vi "main(Test DQMH modules).vi"() -> ()   [LabVIEW 2018, in "Application.lvlib"] (continued)
        n3888 = Or(x=w8878, y=w8876) -> (x .or. y?=w8877:bool)
        n3889 = case shown="False" w8877 {
          tunnel: [w8906 _] -> w8888
          tunnel: w8885 -> [w8905 _]
          frame False {
            w8894 = T9 {"command"="", "data"=variant} ("element")
            w8893 = "MEAS.mux6_1"
            n3890 = To Variant(anything=T2."mux6_1_channel6_2" ("mux6_1(3wires)_encode")) -> (Variant=w8901:variant)
            n3891 = To Variant(anything=T2."mux6_1_channel6_3" ("mux6_1(3wires)_encode")) -> (Variant=w8903:variant)
            n3892 = Bundle By Name(cluster=w8894, "command"=w8893, "data"=w8901) -> (w8900:T9)
            n3893 = Bundle By Name(cluster=w8894, "command"=w8893, "data"=w8903) -> (w8899:T9)
            n3894 = Bundle By Name(cluster=w8894, "command"="MEAS.DMM dual read") -> (w8897:T9)
            n3895 = Build Array(w8900, w8899, w8897) -> (w8895:T9[])
            n3896 = Reverse 1D Array(array=w8895) -> (reversed array=w8896:T9[])
            n3897 = for {
              tunnel: [w8912] -> w8906 mode=indexing
              tunnel: w8905 -> [w8911]
              tunnel: w8896 -> [w8910] mode=indexing
              n3898 = Unbundle By Name(w8910) -> ("command"=w8909:string, "data"=w8908:variant)
              n3899 = call "App enquece.vi"("Priority Enquece"=TRUE, "command data"=w8908, "command"=w8909, "queue in"=w8911) -> ("error out"=w8912:errorcluster)  [unwired: 6 in, 1 out]
            }
          }
          frame True {
          }
        }
        n3900 = Merge Errors(w8886, w8888) -> (w8887:errorcluster)
      }
      frame "Test DRV 37" {
        w8921 = 37  # DUT index(1-60)
        n3901 = call "progress string(SubVI).vi"("String 3"=w8922, "String in"=w8923) -> ("String out"=w8924:string)  [unwired: 9 in]
        n3902 = disable-structure shown="LOGGING==TRUE" {
          disable-tunnel: w8922 -> [w8955 _]
          frame condition #0 (active) {
            n3903 = Empty String/Path?(string/path=w8955) -> (empty?=w8957:bool)
            n3904 = Select(t="Quece timeout", s=w8957, f=w8955) -> (s? t:f=w8954:string)
            n3905 = call "string log (SubVI).vi"("state Name"=w8954) -> ()  [unwired: 9 in, 2 out]
          }
          frame condition #1 {
          }
        }
        n3906 = call "FGV DRV stand.vi"() -> ("Sub-Test.DCV"=w8920:bool)  [unwired: 10 in, 1 out]
        n3907 = Not(x=w8920) -> (.not. x?=w8917:bool)
        n3908 = call "FGV Driver Data.vi"("DUT index(1-60)"=w8921) -> ("DUT SC"=w8919:bool)  [unwired: 7 in, 3 out]
        n3909 = Or(x=w8919, y=w8917) -> (x .or. y?=w8918:bool)
        n3910 = case shown="False" w8918 {
          tunnel: [w8947 _] -> w8929
          tunnel: w8926 -> [w8946 _]
          frame False {
            w8935 = T9 {"command"="", "data"=variant} ("element")
            w8934 = "MEAS.mux6_1"
            n3911 = To Variant(anything=T2."mux6_1_channel1_3" ("mux6_1(3wires)_encode")) -> (Variant=w8944:variant)
            n3912 = To Variant(anything=T2."mux6-1_channel1_2" ("mux6_1(3wires)_encode")) -> (Variant=w8942:variant)
            n3913 = Bundle By Name(cluster=w8935, "command"=w8934, "data"=w8942) -> (w8941:T9)
            n3914 = Bundle By Name(cluster=w8935, "command"=w8934, "data"=w8944) -> (w8940:T9)
            n3915 = Bundle By Name(cluster=w8935, "command"="MEAS.DMM dual read") -> (w8938:T9)
            n3916 = Build Array(w8941, w8940, w8938) -> (w8936:T9[])
            n3917 = Reverse 1D Array(array=w8936) -> (reversed array=w8937:T9[])
            n3918 = for {
              tunnel: [w8953] -> w8947 mode=indexing
              tunnel: w8946 -> [w8952]
              tunnel: w8937 -> [w8951] mode=indexing
              n3919 = Unbundle By Name(w8951) -> ("command"=w8950:string, "data"=w8949:variant)
              n3920 = call "App enquece.vi"("Priority Enquece"=TRUE, "command data"=w8949, "command"=w8950, "queue in"=w8952) -> ("error out"=w8953:errorcluster)  [unwired: 6 in, 1 out]
            }
          }
          frame True {
          }
        }
        n3921 = Merge Errors(w8927, w8929) -> (w8928:errorcluster)
      }
      frame "Test DRV 38" {
        w8963 = 38  # DUT index(1-60)
        n3922 = disable-structure shown="LOGGING==TRUE" {
          disable-tunnel: w8964 -> [w8996 _]
          frame condition #0 (active) {
            n3923 = Empty String/Path?(string/path=w8996) -> (empty?=w8998:bool)
            n3924 = Select(t="Quece timeout", s=w8998, f=w8996) -> (s? t:f=w8995:string)
            n3925 = call "string log (SubVI).vi"("state Name"=w8995) -> ()  [unwired: 9 in, 2 out]
          }
          frame condition #1 {
          }
        }
        n3926 = call "progress string(SubVI).vi"("String 3"=w8964, "String in"=w8965) -> ("String out"=w8966:string)  [unwired: 9 in]
        n3927 = call "FGV DRV stand.vi"() -> ("Sub-Test.DCV"=w8961:bool)  [unwired: 10 in, 1 out]
        n3928 = call "FGV Driver Data.vi"("DUT index(1-60)"=w8963) -> ("DUT SC"=w8960:bool)  [unwired: 7 in, 3 out]
        n3929 = Not(x=w8961) -> (.not. x?=w8958:bool)
        n3930 = Or(x=w8960, y=w8958) -> (x .or. y?=w8959:bool)
        n3931 = case shown="False" w8959 {
          tunnel: [w8988 _] -> w8970
          tunnel: w8968 -> [w8987 _]
          frame False {
            w8976 = T9 {"command"="", "data"=variant} ("element")
            w8975 = "MEAS.mux6_1"
            n3932 = To Variant(anything=T2."mux6_1_channel2_2" ("mux6_1(3wires)_encode")) -> (Variant=w8983:variant)
            n3933 = To Variant(anything=T2."mux6_1_channel2_3" ("mux6_1(3wires)_encode")) -> (Variant=w8985:variant)
            n3934 = Bundle By Name(cluster=w8976, "command"=w8975, "data"=w8983) -> (w8982:T9)
            n3935 = Bundle By Name(cluster=w8976, "command"=w8975, "data"=w8985) -> (w8981:T9)
            n3936 = Bundle By Name(cluster=w8976, "command"="MEAS.DMM dual read") -> (w8979:T9)
            n3937 = Build Array(w8982, w8981, w8979) -> (w8977:T9[])
            n3938 = Reverse 1D Array(array=w8977) -> (reversed array=w8978:T9[])
            n3939 = for {
              tunnel: [w8994] -> w8988 mode=indexing
              tunnel: w8987 -> [w8993]
              tunnel: w8978 -> [w8992] mode=indexing
              n3940 = Unbundle By Name(w8992) -> ("command"=w8991:string, "data"=w8990:variant)
              n3941 = call "App enquece.vi"("Priority Enquece"=TRUE, "command data"=w8990, "command"=w8991, "queue in"=w8993) -> ("error out"=w8994:errorcluster)  [unwired: 6 in, 1 out]
            }
          }
          frame True {
          }
        }
        n3942 = Merge Errors(w8969, w8970) -> (w8962:errorcluster)
      }
      frame "Test DRV 39" {
        w9004 = 39  # DUT index(1-60)
        n3943 = disable-structure shown="LOGGING==TRUE" {
          disable-tunnel: w9005 -> [w9037 _]
          frame condition #0 (active) {
            n3944 = Empty String/Path?(string/path=w9037) -> (empty?=w9039:bool)
            n3945 = Select(t="Quece timeout", s=w9039, f=w9037) -> (s? t:f=w9036:string)
            n3946 = call "string log (SubVI).vi"("state Name"=w9036) -> ()  [unwired: 9 in, 2 out]
          }
          frame condition #1 {
          }
        }
        n3947 = call "progress string(SubVI).vi"("String 3"=w9005, "String in"=w9006) -> ("String out"=w9007:string)  [unwired: 9 in]
        n3948 = call "FGV DRV stand.vi"() -> ("Sub-Test.DCV"=w9003:bool)  [unwired: 10 in, 1 out]
        n3949 = call "FGV Driver Data.vi"("DUT index(1-60)"=w9004) -> ("DUT SC"=w9002:bool)  [unwired: 7 in, 3 out]
        n3950 = Not(x=w9003) -> (.not. x?=w9000:bool)
        n3951 = Or(x=w9002, y=w9000) -> (x .or. y?=w9001:bool)
        n3952 = case shown="False" w9001 {
          tunnel: [w9029 _] -> w9011
          tunnel: w9009 -> [w9028 _]
          frame False {
            w9017 = T9 {"command"="", "data"=variant} ("element")
            w9016 = "MEAS.mux6_1"
            n3953 = To Variant(anything=T2."mux6_1_channel3_3" ("mux6_1(3wires)_encode")) -> (Variant=w9026:variant)
            n3954 = To Variant(anything=T2."mux6_1_channel3_2" ("mux6_1(3wires)_encode")) -> (Variant=w9024:variant)
            n3955 = Bundle By Name(cluster=w9017, "command"=w9016, "data"=w9024) -> (w9023:T9)
            n3956 = Bundle By Name(cluster=w9017, "command"=w9016, "data"=w9026) -> (w9022:T9)
            n3957 = Bundle By Name(cluster=w9017, "command"="MEAS.DMM dual read") -> (w9020:T9)
            n3958 = Build Array(w9023, w9022, w9020) -> (w9018:T9[])
            n3959 = Reverse 1D Array(array=w9018) -> (reversed array=w9019:T9[])
            n3960 = for {
              tunnel: [w9035] -> w9029 mode=indexing
              tunnel: w9028 -> [w9034]
              tunnel: w9019 -> [w9033] mode=indexing
              n3961 = Unbundle By Name(w9033) -> ("command"=w9032:string, "data"=w9031:variant)
              n3962 = call "App enquece.vi"("Priority Enquece"=TRUE, "command data"=w9031, "command"=w9032, "queue in"=w9034) -> ("error out"=w9035:errorcluster)  [unwired: 6 in, 1 out]
            }
          }
          frame True {
          }
        }
        n3963 = Merge Errors(w9010, w9011) -> (w8999:errorcluster)
      }
      frame "Test DRV 40" {
        w9044 = 40  # DUT index(1-60)
        n3964 = disable-structure shown="LOGGING==TRUE" {
          disable-tunnel: w9045 -> [w9078 _]
          frame condition #0 (active) {
            n3965 = Empty String/Path?(string/path=w9078) -> (empty?=w9080:bool)
            n3966 = Select(t="Quece timeout", s=w9080, f=w9078) -> (s? t:f=w9077:string)
            n3967 = call "string log (SubVI).vi"("state Name"=w9077) -> ()  [unwired: 9 in, 2 out]
          }
          frame condition #1 {
          }
        }
        n3968 = call "progress string(SubVI).vi"("String 3"=w9045, "String in"=w9046) -> ("String out"=w9047:string)  [unwired: 9 in]
        n3969 = call "FGV DRV stand.vi"() -> ("Sub-Test.DCV"=w9043:bool)  [unwired: 10 in, 1 out]
        n3970 = call "FGV Driver Data.vi"("DUT index(1-60)"=w9044) -> ("DUT SC"=w9042:bool)  [unwired: 7 in, 3 out]
        n3971 = Not(x=w9043) -> (.not. x?=w9040:bool)
        n3972 = Or(x=w9042, y=w9040) -> (x .or. y?=w9041:bool)
        n3973 = case shown="False" w9041 {
          tunnel: [w9070 _] -> w9052
          tunnel: w9049 -> [w9069 _]
          frame False {
            w9058 = T9 {"command"="", "data"=variant} ("element")
            w9057 = "MEAS.mux6_1"
            n3974 = To Variant(anything=T2."mux6_1_channel4_3" ("mux6_1(3wires)_encode")) -> (Variant=w9067:variant)
            n3975 = To Variant(anything=T2."mux6_1_channel4_2" ("mux6_1(3wires)_encode")) -> (Variant=w9065:variant)
            n3976 = Bundle By Name(cluster=w9058, "command"=w9057, "data"=w9065) -> (w9064:T9)
            n3977 = Bundle By Name(cluster=w9058, "command"=w9057, "data"=w9067) -> (w9063:T9)
            n3978 = Bundle By Name(cluster=w9058, "command"="MEAS.DMM dual read") -> (w9061:T9)
            n3979 = Build Array(w9064, w9063, w9061) -> (w9059:T9[])
            n3980 = Reverse 1D Array(array=w9059) -> (reversed array=w9060:T9[])
            n3981 = for {
              tunnel: [w9076] -> w9070 mode=indexing
              tunnel: w9069 -> [w9075]
              tunnel: w9060 -> [w9074] mode=indexing
              n3982 = Unbundle By Name(w9074) -> ("command"=w9073:string, "data"=w9072:variant)
              n3983 = call "App enquece.vi"("Priority Enquece"=TRUE, "command data"=w9072, "command"=w9073, "queue in"=w9075) -> ("error out"=w9076:errorcluster)  [unwired: 6 in, 1 out]
            }
          }
          frame True {
          }
        }
        n3984 = Merge Errors(w9050, w9052) -> (w9051:errorcluster)
      }
      frame "Test DRV 41" {
        w9085 = 41  # DUT index(1-60)
        n3985 = disable-structure shown="LOGGING==TRUE" {
          disable-tunnel: w9086 -> [w9119 _]
          frame condition #0 (active) {
            n3986 = Empty String/Path?(string/path=w9119) -> (empty?=w9121:bool)
            n3987 = Select(t="Quece timeout", s=w9121, f=w9119) -> (s? t:f=w9118:string)
            n3988 = call "string log (SubVI).vi"("state Name"=w9118) -> ()  [unwired: 9 in, 2 out]
          }
          frame condition #1 {
          }
        }
        n3989 = call "progress string(SubVI).vi"("String 3"=w9086, "String in"=w9087) -> ("String out"=w9088:string)  [unwired: 9 in]
        n3990 = call "FGV DRV stand.vi"() -> ("Sub-Test.DCV"=w9084:bool)  [unwired: 10 in, 1 out]
        n3991 = call "FGV Driver Data.vi"("DUT index(1-60)"=w9085) -> ("DUT SC"=w9083:bool)  [unwired: 7 in, 3 out]
        n3992 = Not(x=w9084) -> (.not. x?=w9081:bool)
        n3993 = Or(x=w9083, y=w9081) -> (x .or. y?=w9082:bool)
        n3994 = case shown="False" w9082 {
          tunnel: [w9111 _] -> w9093
          tunnel: w9090 -> [w9110 _]
          frame False {
            w9099 = T9 {"command"="", "data"=variant} ("element")
            w9098 = "MEAS.mux6_1"
            n3995 = To Variant(anything=T2."mux6_1_channel5_3" ("mux6_1(3wires)_encode")) -> (Variant=w9108:variant)
            n3996 = To Variant(anything=T2."mux6_1_channel5_2" ("mux6_1(3wires)_encode")) -> (Variant=w9106:variant)
            n3997 = Bundle By Name(cluster=w9099, "command"=w9098, "data"=w9106) -> (w9105:T9)
            n3998 = Bundle By Name(cluster=w9099, "command"=w9098, "data"=w9108) -> (w9104:T9)
            n3999 = Bundle By Name(cluster=w9099, "command"="MEAS.DMM dual read") -> (w9102:T9)
            n4000 = Build Array(w9105, w9104, w9102) -> (w9100:T9[])
            n4001 = Reverse 1D Array(array=w9100) -> (reversed array=w9101:T9[])
            n4002 = for {
              tunnel: [w9117] -> w9111 mode=indexing
              tunnel: w9110 -> [w9116]
              tunnel: w9101 -> [w9115] mode=indexing
              n4003 = Unbundle By Name(w9115) -> ("command"=w9114:string, "data"=w9113:variant)
              n4004 = call "App enquece.vi"("Priority Enquece"=TRUE, "command data"=w9113, "command"=w9114, "queue in"=w9116) -> ("error out"=w9117:errorcluster)  [unwired: 6 in, 1 out]
            }
          }
          frame True {
          }
        }
        n4005 = Merge Errors(w9091, w9093) -> (w9092:errorcluster)
      }
      frame "Test DRV 42" {
        w9126 = 42  # DUT index(1-60)
        n4006 = disable-structure shown="LOGGING==TRUE" {
          disable-tunnel: w9127 -> [w9160 _]
          frame condition #0 (active) {
            n4007 = Empty String/Path?(string/path=w9160) -> (empty?=w9162:bool)
            n4008 = Select(t="Quece timeout", s=w9162, f=w9160) -> (s? t:f=w9159:string)
            n4009 = call "string log (SubVI).vi"("state Name"=w9159) -> ()  [unwired: 9 in, 2 out]
          }
          frame condition #1 {
          }
        }
        n4010 = call "progress string(SubVI).vi"("String 3"=w9127, "String in"=w9128) -> ("String out"=w9129:string)  [unwired: 9 in]
        n4011 = call "FGV DRV stand.vi"() -> ("Sub-Test.DCV"=w9125:bool)  [unwired: 10 in, 1 out]
        n4012 = call "FGV Driver Data.vi"("DUT index(1-60)"=w9126) -> ("DUT SC"=w9124:bool)  [unwired: 7 in, 3 out]
        n4013 = Not(x=w9125) -> (.not. x?=w9122:bool)
        n4014 = Or(x=w9124, y=w9122) -> (x .or. y?=w9123:bool)
        n4015 = case shown="False" w9123 {
          tunnel: [w9152 _] -> w9134
          tunnel: w9131 -> [w9151 _]
          frame False {
            w9140 = T9 {"command"="", "data"=variant} ("element")
            w9139 = "MEAS.mux6_1"
            n4016 = To Variant(anything=T2."mux6_1_channel6_3" ("mux6_1(3wires)_encode")) -> (Variant=w9149:variant)
            n4017 = To Variant(anything=T2."mux6_1_channel6_2" ("mux6_1(3wires)_encode")) -> (Variant=w9147:variant)
            n4018 = Bundle By Name(cluster=w9140, "command"=w9139, "data"=w9147) -> (w9146:T9)
            n4019 = Bundle By Name(cluster=w9140, "command"=w9139, "data"=w9149) -> (w9145:T9)
            n4020 = Bundle By Name(cluster=w9140, "command"="MEAS.DMM dual read") -> (w9143:T9)
            n4021 = Build Array(w9146, w9145, w9143) -> (w9141:T9[])
            n4022 = Reverse 1D Array(array=w9141) -> (reversed array=w9142:T9[])
            n4023 = for {
              tunnel: [w9158] -> w9152 mode=indexing
              tunnel: w9151 -> [w9153]
              tunnel: w9142 -> [w9154] mode=indexing
              n4024 = Unbundle By Name(w9154) -> ("command"=w9157:string, "data"=w9156:variant)
              n4025 = call "App enquece.vi"("Priority Enquece"=TRUE, "command data"=w9156, "command"=w9157, "queue in"=w9153) -> ("error out"=w9158:errorcluster)  [unwired: 6 in, 1 out]
            }
          }
          frame True {
          }
        }
        n4026 = Merge Errors(w9132, w9134) -> (w9133:errorcluster)
      }
      frame "Test DRV 43" {
        w9167 = 43  # DUT index(1-60)
        n4027 = disable-structure shown="LOGGING==TRUE" {
          disable-tunnel: w9168 -> [w9201 _]
          frame condition #0 (active) {
            n4028 = Empty String/Path?(string/path=w9201) -> (empty?=w9203:bool)
            n4029 = Select(t="Quece timeout", s=w9203, f=w9201) -> (s? t:f=w9200:string)
            n4030 = call "string log (SubVI).vi"("state Name"=w9200) -> ()  [unwired: 9 in, 2 out]
          }
          frame condition #1 {
          }
        }
        n4031 = call "progress string(SubVI).vi"("String 3"=w9168, "String in"=w9169) -> ("String out"=w9170:string)  [unwired: 9 in]
        n4032 = call "FGV DRV stand.vi"() -> ("Sub-Test.DCV"=w9166:bool)  [unwired: 10 in, 1 out]
        n4033 = call "FGV Driver Data.vi"("DUT index(1-60)"=w9167) -> ("DUT SC"=w9165:bool)  [unwired: 7 in, 3 out]
        n4034 = Not(x=w9166) -> (.not. x?=w9163:bool)
        n4035 = Or(x=w9165, y=w9163) -> (x .or. y?=w9164:bool)
        n4036 = case shown="False" w9164 {
          tunnel: [w9193 _] -> w9175
          tunnel: w9172 -> [w9192 _]
          frame False {
            w9181 = T9 {"command"="", "data"=variant} ("element")
            w9180 = "MEAS.mux6_1"
            n4037 = To Variant(anything=T2."mux6_1_channel1_3" ("mux6_1(3wires)_encode")) -> (Variant=w9190:variant)
            n4038 = To Variant(anything=T2."mux6-1_channel1_2" ("mux6_1(3wires)_encode")) -> (Variant=w9188:variant)
            n4039 = Bundle By Name(cluster=w9181, "command"=w9180, "data"=w9188) -> (w9187:T9)
            n4040 = Bundle By Name(cluster=w9181, "command"=w9180, "data"=w9190) -> (w9186:T9)
            n4041 = Bundle By Name(cluster=w9181, "command"="MEAS.DMM dual read") -> (w9184:T9)
            n4042 = Build Array(w9187, w9186, w9184) -> (w9182:T9[])
            n4043 = Reverse 1D Array(array=w9182) -> (reversed array=w9183:T9[])
            n4044 = for {
              tunnel: [w9199] -> w9193 mode=indexing
              tunnel: w9192 -> [w9198]
              tunnel: w9183 -> [w9197] mode=indexing
              n4045 = Unbundle By Name(w9197) -> ("command"=w9196:string, "data"=w9195:variant)
              n4046 = call "App enquece.vi"("Priority Enquece"=TRUE, "command data"=w9195, "command"=w9196, "queue in"=w9198) -> ("error out"=w9199:errorcluster)  [unwired: 6 in, 1 out]
            }
          }
          frame True {
          }
        }
        n4047 = Merge Errors(w9173, w9175) -> (w9174:errorcluster)
      }
      frame "Test DRV 44" {
        w9208 = 44  # DUT index(1-60)
        n4048 = disable-structure shown="LOGGING==TRUE" {
          disable-tunnel: w9209 -> [w9242 _]
          frame condition #0 (active) {
            n4049 = Empty String/Path?(string/path=w9242) -> (empty?=w9244:bool)
            n4050 = Select(t="Quece timeout", s=w9244, f=w9242) -> (s? t:f=w9241:string)
            n4051 = call "string log (SubVI).vi"("state Name"=w9241) -> ()  [unwired: 9 in, 2 out]
          }
          frame condition #1 {
          }
        }
        n4052 = call "progress string(SubVI).vi"("String 3"=w9209, "String in"=w9210) -> ("String out"=w9211:string)  [unwired: 9 in]
        n4053 = call "FGV DRV stand.vi"() -> ("Sub-Test.DCV"=w9207:bool)  [unwired: 10 in, 1 out]
        n4054 = call "FGV Driver Data.vi"("DUT index(1-60)"=w9208) -> ("DUT SC"=w9206:bool)  [unwired: 7 in, 3 out]
        n4055 = Not(x=w9207) -> (.not. x?=w9204:bool)
        n4056 = Or(x=w9206, y=w9204) -> (x .or. y?=w9205:bool)
        n4057 = case shown="False" w9205 {
          tunnel: [w9234 _] -> w9216
          tunnel: w9213 -> [w9233 _]
          frame False {
            w9222 = T9 {"command"="", "data"=variant} ("element")
            w9221 = "MEAS.mux6_1"
            n4058 = To Variant(anything=T2."mux6_1_channel2_3" ("mux6_1(3wires)_encode")) -> (Variant=w9231:variant)
            n4059 = To Variant(anything=T2."mux6_1_channel2_2" ("mux6_1(3wires)_encode")) -> (Variant=w9229:variant)
            n4060 = Bundle By Name(cluster=w9222, "command"=w9221, "data"=w9229) -> (w9228:T9)
            n4061 = Bundle By Name(cluster=w9222, "command"=w9221, "data"=w9231) -> (w9227:T9)
            n4062 = Bundle By Name(cluster=w9222, "command"="MEAS.DMM dual read") -> (w9225:T9)
            n4063 = Build Array(w9228, w9227, w9225) -> (w9223:T9[])
            n4064 = Reverse 1D Array(array=w9223) -> (reversed array=w9224:T9[])
            n4065 = for {
              tunnel: [w9240] -> w9234 mode=indexing
              tunnel: w9233 -> [w9239]
              tunnel: w9224 -> [w9238] mode=indexing
              n4066 = Unbundle By Name(w9238) -> ("command"=w9237:string, "data"=w9236:variant)
              n4067 = call "App enquece.vi"("Priority Enquece"=TRUE, "command data"=w9236, "command"=w9237, "queue in"=w9239) -> ("error out"=w9240:errorcluster)  [unwired: 6 in, 1 out]
            }
          }
          frame True {
          }
        }
        n4068 = Merge Errors(w9214, w9216) -> (w9215:errorcluster)
      }
      frame "Test DRV 45" {
        w9249 = 45  # DUT index(1-60)
        n4069 = disable-structure shown="LOGGING==TRUE" {
          disable-tunnel: w9250 -> [w9283 _]
          frame condition #0 (active) {
            n4070 = Empty String/Path?(string/path=w9283) -> (empty?=w9285:bool)
            n4071 = Select(t="Quece timeout", s=w9285, f=w9283) -> (s? t:f=w9282:string)
            n4072 = call "string log (SubVI).vi"("state Name"=w9282) -> ()  [unwired: 9 in, 2 out]
          }
          frame condition #1 {
          }
        }
        n4073 = call "progress string(SubVI).vi"("String 3"=w9250, "String in"=w9251) -> ("String out"=w9252:string)  [unwired: 9 in]
        n4074 = call "FGV DRV stand.vi"() -> ("Sub-Test.DCV"=w9248:bool)  [unwired: 10 in, 1 out]
        n4075 = call "FGV Driver Data.vi"("DUT index(1-60)"=w9249) -> ("DUT SC"=w9247:bool)  [unwired: 7 in, 3 out]
        n4076 = Not(x=w9248) -> (.not. x?=w9245:bool)
        n4077 = Or(x=w9247, y=w9245) -> (x .or. y?=w9246:bool)
        n4078 = case shown="False" w9246 {
          tunnel: [w9275 _] -> w9257
          tunnel: w9254 -> [w9274 _]
          frame False {
            w9263 = T9 {"command"="", "data"=variant} ("element")
            w9262 = "MEAS.mux6_1"
            n4079 = To Variant(anything=T2."mux6_1_channel3_3" ("mux6_1(3wires)_encode")) -> (Variant=w9272:variant)
            n4080 = To Variant(anything=T2."mux6_1_channel3_2" ("mux6_1(3wires)_encode")) -> (Variant=w9270:variant)
            n4081 = Bundle By Name(cluster=w9263, "command"=w9262, "data"=w9270) -> (w9269:T9)
            n4082 = Bundle By Name(cluster=w9263, "command"=w9262, "data"=w9272) -> (w9268:T9)
            n4083 = Bundle By Name(cluster=w9263, "command"="MEAS.DMM dual read") -> (w9266:T9)
            n4084 = Build Array(w9269, w9268, w9266) -> (w9264:T9[])
            n4085 = Reverse 1D Array(array=w9264) -> (reversed array=w9265:T9[])
            n4086 = for {
              tunnel: [w9281] -> w9275 mode=indexing
              tunnel: w9274 -> [w9280]
              tunnel: w9265 -> [w9279] mode=indexing
              n4087 = Unbundle By Name(w9279) -> ("command"=w9278:string, "data"=w9277:variant)
              n4088 = call "App enquece.vi"("Priority Enquece"=TRUE, "command data"=w9277, "command"=w9278, "queue in"=w9280) -> ("error out"=w9281:errorcluster)  [unwired: 6 in, 1 out]
            }
          }
          frame True {
          }
        }
        n4089 = Merge Errors(w9255, w9257) -> (w9256:errorcluster)
      }
      frame "Test DRV 46" {
        w9290 = 46  # DUT index(1-60)
        n4090 = disable-structure shown="LOGGING==TRUE" {
          disable-tunnel: w9291 -> [w9324 _]
          frame condition #0 (active) {
            n4091 = Empty String/Path?(string/path=w9324) -> (empty?=w9326:bool)
            n4092 = Select(t="Quece timeout", s=w9326, f=w9324) -> (s? t:f=w9323:string)
            n4093 = call "string log (SubVI).vi"("state Name"=w9323) -> ()  [unwired: 9 in, 2 out]
          }
          frame condition #1 {
          }
        }
        n4094 = call "progress string(SubVI).vi"("String 3"=w9291, "String in"=w9292) -> ("String out"=w9293:string)  [unwired: 9 in]
        n4095 = call "FGV DRV stand.vi"() -> ("Sub-Test.DCV"=w9289:bool)  [unwired: 10 in, 1 out]
        n4096 = call "FGV Driver Data.vi"("DUT index(1-60)"=w9290) -> ("DUT SC"=w9288:bool)  [unwired: 7 in, 3 out]
        n4097 = Not(x=w9289) -> (.not. x?=w9286:bool)
        n4098 = Or(x=w9288, y=w9286) -> (x .or. y?=w9287:bool)
        n4099 = case shown="False" w9287 {
          tunnel: [w9316 _] -> w9298
          tunnel: w9295 -> [w9315 _]
          frame False {
            w9304 = T9 {"command"="", "data"=variant} ("element")
            w9303 = "MEAS.mux6_1"
            n4100 = To Variant(anything=T2."mux6_1_channel4_3" ("mux6_1(3wires)_encode")) -> (Variant=w9313:variant)
            n4101 = To Variant(anything=T2."mux6_1_channel4_2" ("mux6_1(3wires)_encode")) -> (Variant=w9311:variant)
            n4102 = Bundle By Name(cluster=w9304, "command"=w9303, "data"=w9311) -> (w9310:T9)
            n4103 = Bundle By Name(cluster=w9304, "command"=w9303, "data"=w9313) -> (w9309:T9)
            n4104 = Bundle By Name(cluster=w9304, "command"="MEAS.DMM dual read") -> (w9307:T9)
            n4105 = Build Array(w9310, w9309, w9307) -> (w9305:T9[])
            n4106 = Reverse 1D Array(array=w9305) -> (reversed array=w9306:T9[])
            n4107 = for {
              tunnel: [w9322] -> w9316 mode=indexing
              tunnel: w9315 -> [w9321]
              tunnel: w9306 -> [w9320] mode=indexing
              n4108 = Unbundle By Name(w9320) -> ("command"=w9319:string, "data"=w9318:variant)
              n4109 = call "App enquece.vi"("Priority Enquece"=TRUE, "command data"=w9318, "command"=w9319, "queue in"=w9321) -> ("error out"=w9322:errorcluster)  [unwired: 6 in, 1 out]
            }
          }
          frame True {
          }
        }
        n4110 = Merge Errors(w9296, w9298) -> (w9297:errorcluster)
      }
      frame "Test DRV 47" {
        w9331 = 47  # DUT index(1-60)
        n4111 = disable-structure shown="LOGGING==TRUE" {
          disable-tunnel: w9332 -> [w9365 _]
          frame condition #0 (active) {
            n4112 = Empty String/Path?(string/path=w9365) -> (empty?=w9367:bool)
            n4113 = Select(t="Quece timeout", s=w9367, f=w9365) -> (s? t:f=w9364:string)
            n4114 = call "string log (SubVI).vi"("state Name"=w9364) -> ()  [unwired: 9 in, 2 out]
          }
          frame condition #1 {
          }
        }
        n4115 = call "progress string(SubVI).vi"("String 3"=w9332, "String in"=w9333) -> ("String out"=w9334:string)  [unwired: 9 in]
        n4116 = call "FGV DRV stand.vi"() -> ("Sub-Test.DCV"=w9330:bool)  [unwired: 10 in, 1 out]
        n4117 = call "FGV Driver Data.vi"("DUT index(1-60)"=w9331) -> ("DUT SC"=w9329:bool)  [unwired: 7 in, 3 out]
        n4118 = Not(x=w9330) -> (.not. x?=w9327:bool)
        n4119 = Or(x=w9329, y=w9327) -> (x .or. y?=w9328:bool)
        n4120 = case shown="False" w9328 {
          tunnel: [w9357 _] -> w9339
          tunnel: w9336 -> [w9356 _]
          frame False {
            w9345 = T9 {"command"="", "data"=variant} ("element")
            w9344 = "MEAS.mux6_1"
            n4121 = To Variant(anything=T2."mux6_1_channel5_3" ("mux6_1(3wires)_encode")) -> (Variant=w9354:variant)
            n4122 = To Variant(anything=T2."mux6_1_channel5_2" ("mux6_1(3wires)_encode")) -> (Variant=w9352:variant)
            n4123 = Bundle By Name(cluster=w9345, "command"=w9344, "data"=w9352) -> (w9351:T9)
            n4124 = Bundle By Name(cluster=w9345, "command"=w9344, "data"=w9354) -> (w9350:T9)
            n4125 = Bundle By Name(cluster=w9345, "command"="MEAS.DMM dual read") -> (w9348:T9)
            n4126 = Build Array(w9351, w9350, w9348) -> (w9346:T9[])
            n4127 = Reverse 1D Array(array=w9346) -> (reversed array=w9347:T9[])
            n4128 = for {
              tunnel: [w9363] -> w9357 mode=indexing
              tunnel: w9356 -> [w9362]
              tunnel: w9347 -> [w9361] mode=indexing
              n4129 = Unbundle By Name(w9361) -> ("command"=w9360:string, "data"=w9359:variant)
              n4130 = call "App enquece.vi"("Priority Enquece"=TRUE, "command data"=w9359, "command"=w9360, "queue in"=w9362) -> ("error out"=w9363:errorcluster)  [unwired: 6 in, 1 out]
            }
          }
          frame True {
          }
        }
        n4131 = Merge Errors(w9337, w9339) -> (w9338:errorcluster)
      }
      frame "Test DRV 48" {
        w9372 = 48  # DUT index(1-60)
        n4132 = disable-structure shown="LOGGING==TRUE" {
          disable-tunnel: w9373 -> [w9406 _]
          frame condition #0 (active) {
            n4133 = Empty String/Path?(string/path=w9406) -> (empty?=w9408:bool)
            n4134 = Select(t="Quece timeout", s=w9408, f=w9406) -> (s? t:f=w9405:string)
            n4135 = call "string log (SubVI).vi"("state Name"=w9405) -> ()  [unwired: 9 in, 2 out]
          }
          frame condition #1 {
          }
        }
        n4136 = call "progress string(SubVI).vi"("String 3"=w9373, "String in"=w9374) -> ("String out"=w9375:string)  [unwired: 9 in]
        n4137 = call "FGV DRV stand.vi"() -> ("Sub-Test.DCV"=w9371:bool)  [unwired: 10 in, 1 out]
        n4138 = call "FGV Driver Data.vi"("DUT index(1-60)"=w9372) -> ("DUT SC"=w9370:bool)  [unwired: 7 in, 3 out]
        n4139 = Not(x=w9371) -> (.not. x?=w9368:bool)
        n4140 = Or(x=w9370, y=w9368) -> (x .or. y?=w9369:bool)
        n4141 = case shown="False" w9369 {
          tunnel: [w9398 _] -> w9380
          tunnel: w9377 -> [w9397 _]
          frame False {
            w9386 = T9 {"command"="", "data"=variant} ("element")
            w9385 = "MEAS.mux6_1"
            n4142 = To Variant(anything=T2."mux6_1_channel6_3" ("mux6_1(3wires)_encode")) -> (Variant=w9395:variant)
            n4143 = To Variant(anything=T2."mux6_1_channel6_2" ("mux6_1(3wires)_encode")) -> (Variant=w9393:variant)
            n4144 = Bundle By Name(cluster=w9386, "command"=w9385, "data"=w9393) -> (w9392:T9)
            n4145 = Bundle By Name(cluster=w9386, "command"=w9385, "data"=w9395) -> (w9391:T9)
            n4146 = Bundle By Name(cluster=w9386, "command"="MEAS.DMM dual read") -> (w9389:T9)
            n4147 = Build Array(w9392, w9391, w9389) -> (w9387:T9[])
            n4148 = Reverse 1D Array(array=w9387) -> (reversed array=w9388:T9[])
            n4149 = for {
              tunnel: [w9404] -> w9398 mode=indexing
              tunnel: w9397 -> [w9403]
              tunnel: w9388 -> [w9402] mode=indexing
              n4150 = Unbundle By Name(w9402) -> ("command"=w9401:string, "data"=w9400:variant)
              n4151 = call "App enquece.vi"("Priority Enquece"=TRUE, "command data"=w9400, "command"=w9401, "queue in"=w9403) -> ("error out"=w9404:errorcluster)  [unwired: 6 in, 1 out]
            }
          }
          frame True {
          }
        }
        n4152 = Merge Errors(w9378, w9380) -> (w9379:errorcluster)
      }
      frame "Test DRV 49" {
        w9413 = 49  # DUT index(1-60)
        n4153 = disable-structure shown="LOGGING==TRUE" {
          disable-tunnel: w9414 -> [w9447 _]
          frame condition #0 (active) {
            n4154 = Empty String/Path?(string/path=w9447) -> (empty?=w9449:bool)
            n4155 = Select(t="Quece timeout", s=w9449, f=w9447) -> (s? t:f=w9446:string)
            n4156 = call "string log (SubVI).vi"("state Name"=w9446) -> ()  [unwired: 9 in, 2 out]
          }
          frame condition #1 {
          }
        }
        n4157 = call "progress string(SubVI).vi"("String 3"=w9414, "String in"=w9415) -> ("String out"=w9416:string)  [unwired: 9 in]
        n4158 = call "FGV DRV stand.vi"() -> ("Sub-Test.DCV"=w9412:bool)  [unwired: 10 in, 1 out]
        n4159 = call "FGV Driver Data.vi"("DUT index(1-60)"=w9413) -> ("DUT SC"=w9411:bool)  [unwired: 7 in, 3 out]
        n4160 = Not(x=w9412) -> (.not. x?=w9409:bool)
        n4161 = Or(x=w9411, y=w9409) -> (x .or. y?=w9410:bool)
        n4162 = case shown="False" w9410 {
          tunnel: [w9439 _] -> w9421
          tunnel: w9418 -> [w9438 _]
          frame False {
            w9427 = T9 {"command"="", "data"=variant} ("element")
            w9426 = "MEAS.mux6_1"
            n4163 = To Variant(anything=T2."mux6_1_channel1_3" ("mux6_1(3wires)_encode")) -> (Variant=w9436:variant)
            n4164 = To Variant(anything=T2."mux6-1_channel1_2" ("mux6_1(3wires)_encode")) -> (Variant=w9434:variant)
            n4165 = Bundle By Name(cluster=w9427, "command"=w9426, "data"=w9434) -> (w9433:T9)
            n4166 = Bundle By Name(cluster=w9427, "command"=w9426, "data"=w9436) -> (w9432:T9)
            n4167 = Bundle By Name(cluster=w9427, "command"="MEAS.DMM dual read") -> (w9430:T9)
            n4168 = Build Array(w9433, w9432, w9430) -> (w9428:T9[])
            n4169 = Reverse 1D Array(array=w9428) -> (reversed array=w9429:T9[])
            n4170 = for {
              tunnel: [w9445] -> w9439 mode=indexing
              tunnel: w9438 -> [w9444]
              tunnel: w9429 -> [w9443] mode=indexing
              n4171 = Unbundle By Name(w9443) -> ("command"=w9442:string, "data"=w9441:variant)
              n4172 = call "App enquece.vi"("Priority Enquece"=TRUE, "command data"=w9441, "command"=w9442, "queue in"=w9444) -> ("error out"=w9445:errorcluster)  [unwired: 6 in, 1 out]
            }
          }
          frame True {
          }
        }
        n4173 = Merge Errors(w9419, w9421) -> (w9420:errorcluster)
      }
      frame "Test DRV 50" {
        w9454 = 50  # DUT index(1-60)
        n4174 = disable-structure shown="LOGGING==TRUE" {
          disable-tunnel: w9455 -> [w9488 _]
          frame condition #0 (active) {
            n4175 = Empty String/Path?(string/path=w9488) -> (empty?=w9490:bool)
            n4176 = Select(t="Quece timeout", s=w9490, f=w9488) -> (s? t:f=w9487:string)
            n4177 = call "string log (SubVI).vi"("state Name"=w9487) -> ()  [unwired: 9 in, 2 out]
          }
          frame condition #1 {
          }
        }
        n4178 = call "progress string(SubVI).vi"("String 3"=w9455, "String in"=w9456) -> ("String out"=w9457:string)  [unwired: 9 in]
        n4179 = call "FGV DRV stand.vi"() -> ("Sub-Test.DCV"=w9453:bool)  [unwired: 10 in, 1 out]
        n4180 = call "FGV Driver Data.vi"("DUT index(1-60)"=w9454) -> ("DUT SC"=w9452:bool)  [unwired: 7 in, 3 out]
        n4181 = Not(x=w9453) -> (.not. x?=w9450:bool)
        n4182 = Or(x=w9452, y=w9450) -> (x .or. y?=w9451:bool)
        n4183 = case shown="False" w9451 {
          tunnel: [w9480 _] -> w9462
          tunnel: w9459 -> [w9467 _]
          frame False {
            w9469 = T9 {"command"="", "data"=variant} ("element")
            w9468 = "MEAS.mux6_1"
            n4184 = To Variant(anything=T2."mux6_1_channel2_3" ("mux6_1(3wires)_encode")) -> (Variant=w9478:variant)
            n4185 = To Variant(anything=T2."mux6_1_channel2_2" ("mux6_1(3wires)_encode")) -> (Variant=w9476:variant)
            n4186 = Bundle By Name(cluster=w9469, "command"=w9468, "data"=w9476) -> (w9475:T9)
            n4187 = Bundle By Name(cluster=w9469, "command"=w9468, "data"=w9478) -> (w9474:T9)
            n4188 = Bundle By Name(cluster=w9469, "command"="MEAS.DMM dual read") -> (w9472:T9)
            n4189 = Build Array(w9475, w9474, w9472) -> (w9470:T9[])
            n4190 = Reverse 1D Array(array=w9470) -> (reversed array=w9471:T9[])
            n4191 = for {
              tunnel: [w9486] -> w9480 mode=indexing
              tunnel: w9467 -> [w9485]
              tunnel: w9471 -> [w9484] mode=indexing
              n4192 = Unbundle By Name(w9484) -> ("command"=w9483:string, "data"=w9482:variant)
              n4193 = call "App enquece.vi"("Priority Enquece"=TRUE, "command data"=w9482, "command"=w9483, "queue in"=w9485) -> ("error out"=w9486:errorcluster)  [unwired: 6 in, 1 out]
            }
          }
          frame True {
          }
        }
        n4194 = Merge Errors(w9460, w9462) -> (w9461:errorcluster)
      }
      frame "Test DRV 51" {
        w9495 = 51  # DUT index(1-60)
        n4195 = disable-structure shown="LOGGING==TRUE" {
          disable-tunnel: w9496 -> [w9529 _]
          frame condition #0 (active) {
            n4196 = Empty String/Path?(string/path=w9529) -> (empty?=w9531:bool)
            n4197 = Select(t="Quece timeout", s=w9531, f=w9529) -> (s? t:f=w9528:string)
            n4198 = call "string log (SubVI).vi"("state Name"=w9528) -> ()  [unwired: 9 in, 2 out]
          }
          frame condition #1 {
          }
        }
        n4199 = call "progress string(SubVI).vi"("String 3"=w9496, "String in"=w9497) -> ("String out"=w9498:string)  [unwired: 9 in]
        n4200 = call "FGV DRV stand.vi"() -> ("Sub-Test.DCV"=w9494:bool)  [unwired: 10 in, 1 out]
        n4201 = call "FGV Driver Data.vi"("DUT index(1-60)"=w9495) -> ("DUT SC"=w9493:bool)  [unwired: 7 in, 3 out]
        n4202 = Not(x=w9494) -> (.not. x?=w9491:bool)
        n4203 = Or(x=w9493, y=w9491) -> (x .or. y?=w9492:bool)
        n4204 = case shown="False" w9492 {
          tunnel: [w9521 _] -> w9503
          tunnel: w9500 -> [w9520 _]
          frame False {
            w9509 = T9 {"command"="", "data"=variant} ("element")
            w9508 = "MEAS.mux6_1"
            n4205 = To Variant(anything=T2."mux6_1_channel3_3" ("mux6_1(3wires)_encode")) -> (Variant=w9518:variant)
            n4206 = To Variant(anything=T2."mux6_1_channel3_2" ("mux6_1(3wires)_encode")) -> (Variant=w9516:variant)
            n4207 = Bundle By Name(cluster=w9509, "command"=w9508, "data"=w9516) -> (w9515:T9)
            n4208 = Bundle By Name(cluster=w9509, "command"=w9508, "data"=w9518) -> (w9514:T9)
            n4209 = Bundle By Name(cluster=w9509, "command"="MEAS.DMM dual read") -> (w9512:T9)
            n4210 = Build Array(w9515, w9514, w9512) -> (w9510:T9[])
            n4211 = Reverse 1D Array(array=w9510) -> (reversed array=w9511:T9[])
            n4212 = for {
              tunnel: [w9527] -> w9521 mode=indexing
              tunnel: w9520 -> [w9526]
              tunnel: w9511 -> [w9525] mode=indexing
              n4213 = Unbundle By Name(w9525) -> ("command"=w9524:string, "data"=w9523:variant)
              n4214 = call "App enquece.vi"("Priority Enquece"=TRUE, "command data"=w9523, "command"=w9524, "queue in"=w9526) -> ("error out"=w9527:errorcluster)  [unwired: 6 in, 1 out]
            }
          }
          frame True {
          }
        }
        n4215 = Merge Errors(w9501, w9503) -> (w9502:errorcluster)
      }
      frame "Test DRV 52" {
        w9536 = 52  # DUT index(1-60)
        n4216 = disable-structure shown="LOGGING==TRUE" {
          disable-tunnel: w9537 -> [w9570 _]
          frame condition #0 (active) {
            n4217 = Empty String/Path?(string/path=w9570) -> (empty?=w9572:bool)
            n4218 = Select(t="Quece timeout", s=w9572, f=w9570) -> (s? t:f=w9569:string)
            n4219 = call "string log (SubVI).vi"("state Name"=w9569) -> ()  [unwired: 9 in, 2 out]
          }
          frame condition #1 {
          }
        }
        n4220 = call "progress string(SubVI).vi"("String 3"=w9537, "String in"=w9538) -> ("String out"=w9539:string)  [unwired: 9 in]
        n4221 = call "FGV DRV stand.vi"() -> ("Sub-Test.DCV"=w9535:bool)  [unwired: 10 in, 1 out]
        n4222 = call "FGV Driver Data.vi"("DUT index(1-60)"=w9536) -> ("DUT SC"=w9534:bool)  [unwired: 7 in, 3 out]
        n4223 = Not(x=w9535) -> (.not. x?=w9532:bool)
        n4224 = Or(x=w9534, y=w9532) -> (x .or. y?=w9533:bool)
        n4225 = case shown="False" w9533 {
          tunnel: [w9562 _] -> w9544
          tunnel: w9541 -> [w9561 _]
          frame False {
            w9550 = T9 {"command"="", "data"=variant} ("element")
            w9549 = "MEAS.mux6_1"
            n4226 = To Variant(anything=T2."mux6_1_channel4_3" ("mux6_1(3wires)_encode")) -> (Variant=w9559:variant)
            n4227 = To Variant(anything=T2."mux6_1_channel4_2" ("mux6_1(3wires)_encode")) -> (Variant=w9557:variant)
            n4228 = Bundle By Name(cluster=w9550, "command"=w9549, "data"=w9557) -> (w9556:T9)
            n4229 = Bundle By Name(cluster=w9550, "command"=w9549, "data"=w9559) -> (w9555:T9)
            n4230 = Bundle By Name(cluster=w9550, "command"="MEAS.DMM dual read") -> (w9553:T9)
            n4231 = Build Array(w9556, w9555, w9553) -> (w9551:T9[])
            n4232 = Reverse 1D Array(array=w9551) -> (reversed array=w9552:T9[])
            n4233 = for {
              tunnel: [w9568] -> w9562 mode=indexing
              tunnel: w9561 -> [w9567]
              tunnel: w9552 -> [w9566] mode=indexing
              n4234 = Unbundle By Name(w9566) -> ("command"=w9565:string, "data"=w9564:variant)
              n4235 = call "App enquece.vi"("Priority Enquece"=TRUE, "command data"=w9564, "command"=w9565, "queue in"=w9567) -> ("error out"=w9568:errorcluster)  [unwired: 6 in, 1 out]
            }
          }
          frame True {
          }
        }
        n4236 = Merge Errors(w9542, w9544) -> (w9543:errorcluster)
      }
      frame "Test DRV 53" {
        w9577 = 53  # DUT index(1-60)
        n4237 = disable-structure shown="LOGGING==TRUE" {
          disable-tunnel: w9578 -> [w9611 _]
          frame condition #0 (active) {
            n4238 = Empty String/Path?(string/path=w9611) -> (empty?=w9613:bool)
            n4239 = Select(t="Quece timeout", s=w9613, f=w9611) -> (s? t:f=w9610:string)
            n4240 = call "string log (SubVI).vi"("state Name"=w9610) -> ()  [unwired: 9 in, 2 out]
          }
          frame condition #1 {
          }
        }
        n4241 = call "progress string(SubVI).vi"("String 3"=w9578, "String in"=w9579) -> ("String out"=w9580:string)  [unwired: 9 in]
        n4242 = call "FGV DRV stand.vi"() -> ("Sub-Test.DCV"=w9576:bool)  [unwired: 10 in, 1 out]
        n4243 = call "FGV Driver Data.vi"("DUT index(1-60)"=w9577) -> ("DUT SC"=w9575:bool)  [unwired: 7 in, 3 out]
        n4244 = Not(x=w9576) -> (.not. x?=w9573:bool)
        n4245 = Or(x=w9575, y=w9573) -> (x .or. y?=w9574:bool)
        n4246 = case shown="False" w9574 {
          tunnel: [w9603 _] -> w9585
          tunnel: w9582 -> [w9602 _]
          frame False {
            w9590 = T9 {"command"="", "data"=variant} ("element")
            w9591 = "MEAS.mux6_1"
            n4247 = To Variant(anything=T2."mux6_1_channel5_3" ("mux6_1(3wires)_encode")) -> (Variant=w9600:variant)
            n4248 = To Variant(anything=T2."mux6_1_channel5_2" ("mux6_1(3wires)_encode")) -> (Variant=w9598:variant)
            n4249 = Bundle By Name(cluster=w9590, "command"=w9591, "data"=w9598) -> (w9597:T9)
            n4250 = Bundle By Name(cluster=w9590, "command"=w9591, "data"=w9600) -> (w9596:T9)
            n4251 = Bundle By Name(cluster=w9590, "command"="MEAS.DMM dual read") -> (w9594:T9)
            n4252 = Build Array(w9597, w9596, w9594) -> (w9592:T9[])
            n4253 = Reverse 1D Array(array=w9592) -> (reversed array=w9593:T9[])
            n4254 = for {
              tunnel: [w9609] -> w9603 mode=indexing
              tunnel: w9602 -> [w9608]
              tunnel: w9593 -> [w9607] mode=indexing
              n4255 = Unbundle By Name(w9607) -> ("command"=w9606:string, "data"=w9605:variant)
              n4256 = call "App enquece.vi"("Priority Enquece"=TRUE, "command data"=w9605, "command"=w9606, "queue in"=w9608) -> ("error out"=w9609:errorcluster)  [unwired: 6 in, 1 out]
            }
          }
          frame True {
          }
        }
        n4257 = Merge Errors(w9583, w9585) -> (w9584:errorcluster)
      }
      frame "Test DRV 54" {
        w9618 = 54  # DUT index(1-60)
        n4258 = disable-structure shown="LOGGING==TRUE" {
          disable-tunnel: w9619 -> [w9652 _]
          frame condition #0 (active) {
            n4259 = Empty String/Path?(string/path=w9652) -> (empty?=w9654:bool)
            n4260 = Select(t="Quece timeout", s=w9654, f=w9652) -> (s? t:f=w9651:string)
            n4261 = call "string log (SubVI).vi"("state Name"=w9651) -> ()  [unwired: 9 in, 2 out]
          }
          frame condition #1 {
          }
        }
        n4262 = call "progress string(SubVI).vi"("String 3"=w9619, "String in"=w9620) -> ("String out"=w9621:string)  [unwired: 9 in]
        n4263 = call "FGV DRV stand.vi"() -> ("Sub-Test.DCV"=w9617:bool)  [unwired: 10 in, 1 out]
        n4264 = call "FGV Driver Data.vi"("DUT index(1-60)"=w9618) -> ("DUT SC"=w9616:bool)  [unwired: 7 in, 3 out]
        n4265 = Not(x=w9617) -> (.not. x?=w9614:bool)
        n4266 = Or(x=w9616, y=w9614) -> (x .or. y?=w9615:bool)
        n4267 = case shown="False" w9615 {
          tunnel: [w9644 _] -> w9626
          tunnel: w9623 -> [w9643 _]
          frame False {
            w9632 = T9 {"command"="", "data"=variant} ("element")
            w9631 = "MEAS.mux6_1"
            n4268 = To Variant(anything=T2."mux6_1_channel6_3" ("mux6_1(3wires)_encode")) -> (Variant=w9641:variant)
            n4269 = To Variant(anything=T2."mux6_1_channel6_2" ("mux6_1(3wires)_encode")) -> (Variant=w9639:variant)
            n4270 = Bundle By Name(cluster=w9632, "command"=w9631, "data"=w9639) -> (w9638:T9)
            n4271 = Bundle By Name(cluster=w9632, "command"=w9631, "data"=w9641) -> (w9637:T9)
            n4272 = Bundle By Name(cluster=w9632, "command"="MEAS.DMM dual read") -> (w9635:T9)
            n4273 = Build Array(w9638, w9637, w9635) -> (w9633:T9[])
            n4274 = Reverse 1D Array(array=w9633) -> (reversed array=w9634:T9[])
            n4275 = for {
              tunnel: [w9650] -> w9644 mode=indexing
              tunnel: w9643 -> [w9649]
              tunnel: w9634 -> [w9648] mode=indexing
              n4276 = Unbundle By Name(w9648) -> ("command"=w9647:string, "data"=w9646:variant)
              n4277 = call "App enquece.vi"("Priority Enquece"=TRUE, "command data"=w9646, "command"=w9647, "queue in"=w9649) -> ("error out"=w9650:errorcluster)  [unwired: 6 in, 1 out]
            }
          }
          frame True {
          }
        }
        n4278 = Merge Errors(w9624, w9626) -> (w9625:errorcluster)
      }
      frame "Test DRV 55" {
        w9660 = 55  # DUT index(1-60)
        n4279 = call "progress string(SubVI).vi"("String 3"=w9659, "String in"=w9661) -> ("String out"=w9662:string)  [unwired: 9 in]
        n4280 = disable-structure shown="LOGGING==TRUE" {
          disable-tunnel: w9659 -> [w9693 _]
          frame condition #0 (active) {
            n4281 = Empty String/Path?(string/path=w9693) -> (empty?=w9695:bool)
            n4282 = Select(t="Quece timeout", s=w9695, f=w9693) -> (s? t:f=w9692:string)
            n4283 = call "string log (SubVI).vi"("state Name"=w9692) -> ()  [unwired: 9 in, 2 out]
          }
          frame condition #1 {
          }
        }
        n4284 = call "FGV DRV stand.vi"() -> ("Sub-Test.DCV"=w9658:bool)  [unwired: 10 in, 1 out]
        n4285 = call "FGV Driver Data.vi"("DUT index(1-60)"=w9660) -> ("DUT SC"=w9657:bool)  [unwired: 7 in, 3 out]
        n4286 = Not(x=w9658) -> (.not. x?=w9655:bool)
        n4287 = Or(x=w9657, y=w9655) -> (x .or. y?=w9656:bool)
        n4288 = case shown="False" w9656 {
          tunnel: [w9685 _] -> w9667
          tunnel: w9664 -> [w9684 _]
          frame False {
            w9673 = T9 {"command"="", "data"=variant} ("element")
            w9672 = "MEAS.mux6_1"
            n4289 = To Variant(anything=T2."mux6_1_channel1_3" ("mux6_1(3wires)_encode")) -> (Variant=w9682:variant)
            n4290 = To Variant(anything=T2."mux6-1_channel1_2" ("mux6_1(3wires)_encode")) -> (Variant=w9680:variant)
            n4291 = Bundle By Name(cluster=w9673, "command"=w9672, "data"=w9680) -> (w9679:T9)
            n4292 = Bundle By Name(cluster=w9673, "command"=w9672, "data"=w9682) -> (w9678:T9)
            n4293 = Bundle By Name(cluster=w9673, "command"="MEAS.DMM dual read") -> (w9676:T9)
            n4294 = Build Array(w9679, w9678, w9676) -> (w9674:T9[])
            n4295 = Reverse 1D Array(array=w9674) -> (reversed array=w9675:T9[])
            n4296 = for {
              tunnel: [w9691] -> w9685 mode=indexing
              tunnel: w9684 -> [w9690]
              tunnel: w9675 -> [w9689] mode=indexing
              n4297 = Unbundle By Name(w9689) -> ("command"=w9688:string, "data"=w9687:variant)
              n4298 = call "App enquece.vi"("Priority Enquece"=TRUE, "command data"=w9687, "command"=w9688, "queue in"=w9690) -> ("error out"=w9691:errorcluster)  [unwired: 6 in, 1 out]
            }
          }
          frame True {
          }
        }
        n4299 = Merge Errors(w9665, w9667) -> (w9666:errorcluster)
      }
      frame "Test DRV 56" {
        w9700 = 56  # DUT index(1-60)
        n4300 = call "progress string(SubVI).vi"("String 3"=w9701, "String in"=w9702) -> ("String out"=w9703:string)  [unwired: 9 in]
        n4301 = disable-structure shown="LOGGING==TRUE" {
          disable-tunnel: w9701 -> [w9734 _]
          frame condition #0 (active) {
            n4302 = Empty String/Path?(string/path=w9734) -> (empty?=w9736:bool)
            n4303 = Select(t="Quece timeout", s=w9736, f=w9734) -> (s? t:f=w9733:string)
            n4304 = call "string log (SubVI).vi"("state Name"=w9733) -> ()  [unwired: 9 in, 2 out]
          }
          frame condition #1 {
          }
        }
        n4305 = call "FGV DRV stand.vi"() -> ("Sub-Test.DCV"=w9699:bool)  [unwired: 10 in, 1 out]
        n4306 = call "FGV Driver Data.vi"("DUT index(1-60)"=w9700) -> ("DUT SC"=w9698:bool)  [unwired: 7 in, 3 out]
        n4307 = Not(x=w9699) -> (.not. x?=w9696:bool)
        n4308 = Or(x=w9698, y=w9696) -> (x .or. y?=w9697:bool)
        n4309 = case shown="False" w9697 {
          tunnel: [w9726 _] -> w9708
          tunnel: w9705 -> [w9725 _]
          frame False {
            w9714 = T9 {"command"="", "data"=variant} ("element")
            w9713 = "MEAS.mux6_1"
            n4310 = To Variant(anything=T2."mux6_1_channel2_3" ("mux6_1(3wires)_encode")) -> (Variant=w9723:variant)
            n4311 = To Variant(anything=T2."mux6_1_channel2_2" ("mux6_1(3wires)_encode")) -> (Variant=w9721:variant)
            n4312 = Bundle By Name(cluster=w9714, "command"=w9713, "data"=w9721) -> (w9720:T9)
            n4313 = Bundle By Name(cluster=w9714, "command"=w9713, "data"=w9723) -> (w9719:T9)
            n4314 = Bundle By Name(cluster=w9714, "command"="MEAS.DMM dual read") -> (w9717:T9)
            n4315 = Build Array(w9720, w9719, w9717) -> (w9715:T9[])
            n4316 = Reverse 1D Array(array=w9715) -> (reversed array=w9716:T9[])
            n4317 = for {
              tunnel: [w9732] -> w9726 mode=indexing
              tunnel: w9725 -> [w9731]
              tunnel: w9716 -> [w9730] mode=indexing
              n4318 = Unbundle By Name(w9730) -> ("command"=w9729:string, "data"=w9728:variant)
              n4319 = call "App enquece.vi"("Priority Enquece"=TRUE, "command data"=w9728, "command"=w9729, "queue in"=w9731) -> ("error out"=w9732:errorcluster)  [unwired: 6 in, 1 out]
            }
          }
          frame True {
          }
        }
        n4320 = Merge Errors(w9706, w9708) -> (w9707:errorcluster)
      }
      frame "Test DRV 57" {
        w9741 = 57  # DUT index(0-59)
        n4321 = disable-structure shown="LOGGING==TRUE" {
          disable-tunnel: w9742 -> [w9775 _]
          frame condition #0 (active) {
            n4322 = Empty String/Path?(string/path=w9775) -> (empty?=w9777:bool)
            n4323 = Select(t="Quece timeout", s=w9777, f=w9775) -> (s? t:f=w9774:string)
            n4324 = call "string log (SubVI).vi"("state Name"=w9774) -> ()  [unwired: 9 in, 2 out]
          }
          frame condition #1 {
          }
        }
        n4325 = call "progress string(SubVI).vi"("String 3"=w9742, "String in"=w9743) -> ("String out"=w9744:string)  [unwired: 9 in]
        n4326 = call "FGV DRV stand.vi"() -> ("Sub-Test.DCV"=w9740:bool)  [unwired: 10 in, 1 out]
        n4327 = call "FGV Driver Data.vi"("DUT index(1-60)"=w9741) -> ("DUT SC"=w9739:bool)  [unwired: 7 in, 3 out]
        n4328 = Not(x=w9740) -> (.not. x?=w9737:bool)
